vi "Read.vi"(7 "length":u16, 8 "error in (no error)":errorcluster, 9 "Start address":string, 10 "Read Type":variant, 11 "MelsecTCP in":refnum<class "InovanceSerialModbusRtu.lvclass">) -> (0 "error out":errorcluster, 2 "Data":variant, 3 "MelsecTCP out":refnum<class "InovanceSerialModbusRtu.lvclass">)   [LabVIEW 2020, in "HslCommunication.lvlib" / "InovanceSerialModbusRtu.lvclass"]
uses:
  InovanceSerialModbusRtu.lvclass
  D:/Git/Labview-Libraries/Libraries/HslCommunication/Abstract PLC Controler/Abstract PLC Controler.lvclass
  EventLogger.lvlibp/1abvi3w/vi.lib/gpm_packages/@cs/event-logger/Source/Composed Log/Types/Log Level.ctl
  Abstract PLC Controler/Abstract PLC Controler.lvclass/Abstract PLC Controler.ctl
  D:/Git/Labview-Libraries/Libraries/HslCommunication/_Dependenciecs/HslCommunication.dll
  _Dependenciecs/HslCommunication.dll
  Read reference.vi
  Abstract PLC Controler/Abstract PLC Controler.lvclass
  <vilib>/Utility/Data Type/NI_Data Type.lvlib
  EventLogger.lvlibp/Logger.lvclass
  EventLogger.lvlibp/1abvi3w/vi.lib/gpm_packages/@cs/event-logger/Source/Composed Log/Composed Log.lvlib
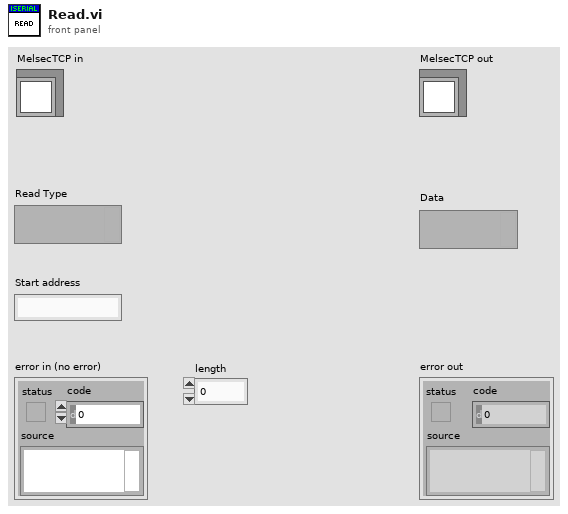
[diagram p1: front panel]
types:
  T1 = typedef "EventLogger.lvlibp/Composed Log.lvlib/Log Level.ctl" = enum16{"Debug", "Info", "Warning", "Error", "Critical"}
  T2 = typedef "NI_Data Type.lvlib/Data Type.ctl" = enum8{"Invalid Type", "Void", "I8", "I16", "I32", "I64", "U8", "U16", "U32", "U64", "Single Float", "Double Float", "Extended Float", "Single Complex", "Double Complex", "Extended Complex", "Enum U8", "Enum U16", "Enum U32", "Enum U64", "Single Float With Unit", "Double Float With Unit", "Extended Float With Unit", "Single Complex with Unit", "Double Complex with Unit", "Extended Complex with Unit", "Boolean", "String", "Path", "Picture", "Tag", "Array", "Cluster", "Variant", "LV Variant", "Waveform", "Timestamp", "Digital Waveform", "Digital Data", "ExpressData", "Refnum", "External Data", "VI", "Poly VI", "LabVIEW Class Instance", "Fixed Point", "Set Collection", "Map Collection"}
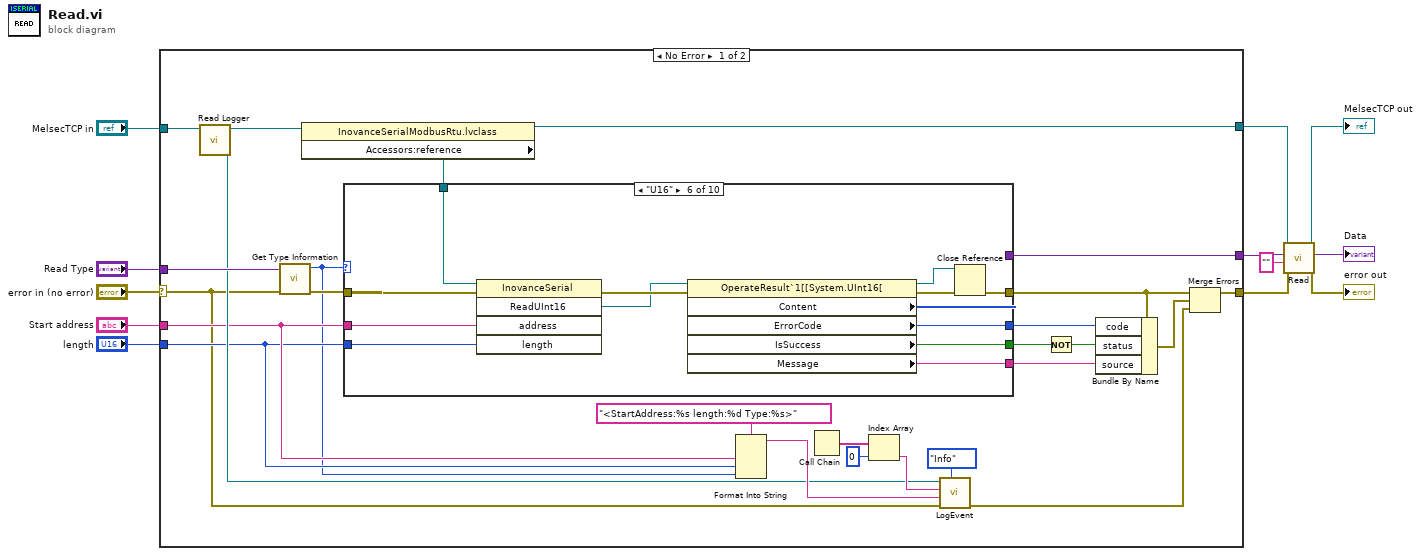
[diagram p0: block diagram]
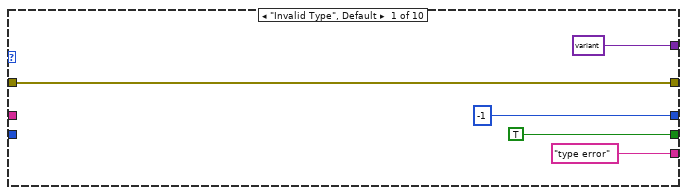
[diagram p2: hidden frame]
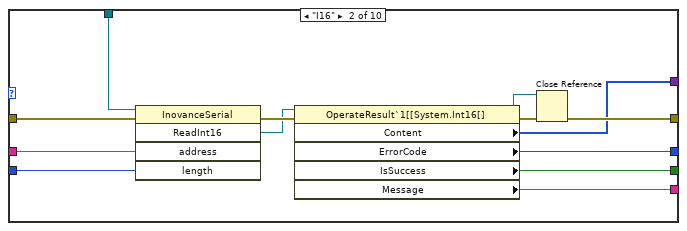
[diagram p3: hidden frame]
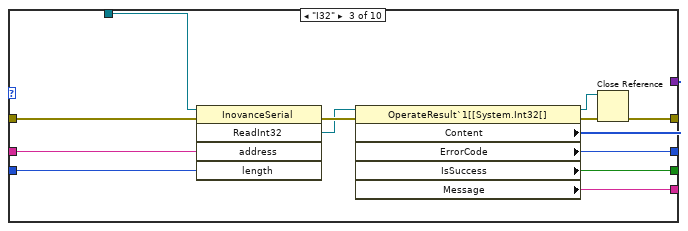
[diagram p4: hidden frame]
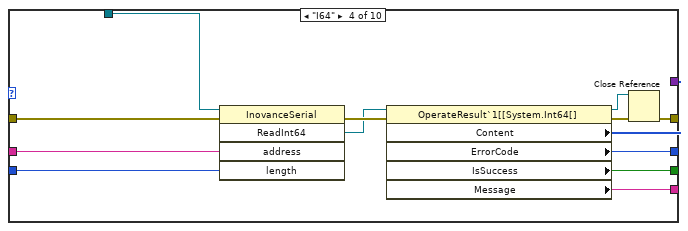
[diagram p5: hidden frame]
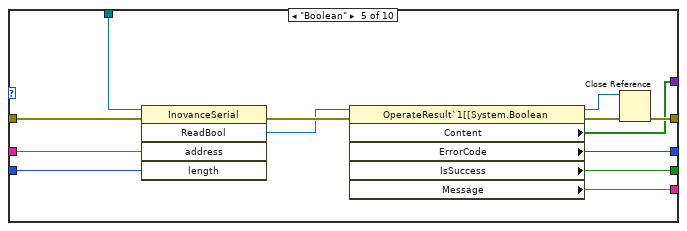
[diagram p6: hidden frame]
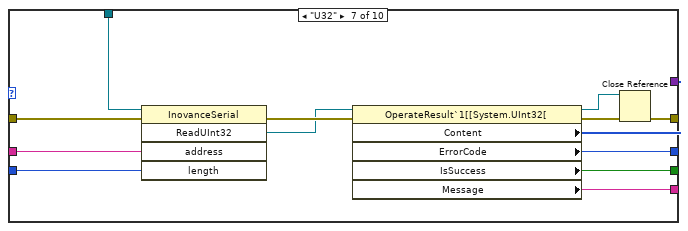
[diagram p7: hidden frame]
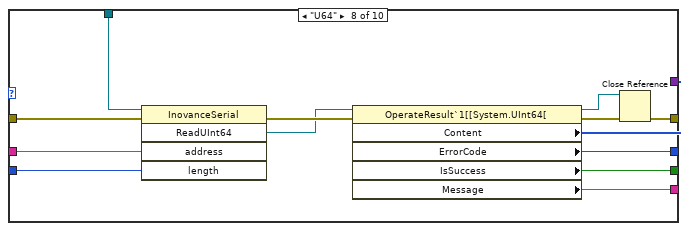
[diagram p8: hidden frame]
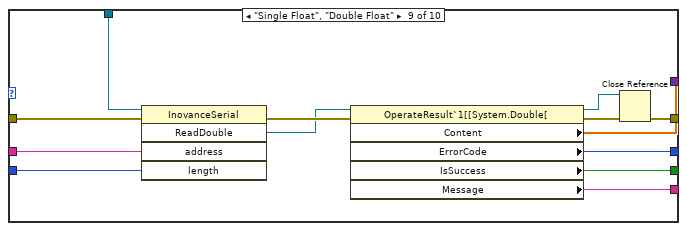
[diagram p9: hidden frame]
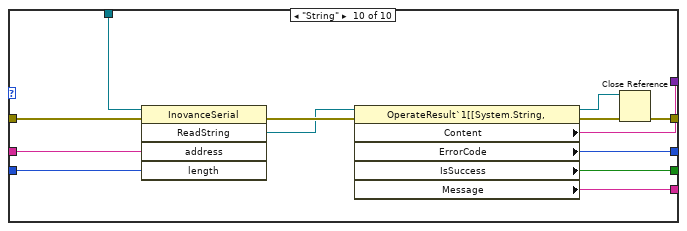
[diagram p10: hidden frame]
diagram:
  n1 = case shown="No Error" "error in (no error)" {
    selector: "error in (no error)" -> [w14 w163]
    tunnel: "MelsecTCP in" -> [w38 w162]
    tunnel: [w29 w162] -> w5
    tunnel: "Start address" -> [w17 _]
    tunnel: [w35 w163] -> w8
    tunnel: [w36 w161] -> w3
    tunnel: "length" -> [w16 _]
    tunnel: "Read Type" -> [w28 w161]
    frame No Error {
      n2 = call "Read Logger.vi"("Abstract PLC Controler in"=w38) -> ("EventLogger.lvlibp:Logger.lvclass"=w19:refnum<class "Logger.lvclass">, "Abstract PLC Controler out"=w20:refnum<class "InovanceSerialModbusRtu.lvclass">)  [unwired: 9 in]
      n3 = call <vilib>:"Get Type Information.vi"("error in (no error)"=w14, "variant"=w28) -> ("error out"=w27:errorcluster, "type"=w15:T2)  [unwired: 5 in, 3 out]
      n4 = property class="InovanceSerialModbusRtu.lvclass"(reference=w20) -> (reference out=w29:refnum<class "InovanceSerialModbusRtu.lvclass">, "Accessors:reference"=w37:refnum<k24>)  [unwired: 1 in, 1 out]
      n5 = case shown="\"U16\"" w15 {
        tunnel: w37 -> [_ w56 w69 w82 w84 w97 w110 w123 w136 w149]
        tunnel: w17 -> [_ w55 w68 w81 w95 w108 w121 w134 w147 w160]
        tunnel: w16 -> [_ w54 w67 w80 w94 w107 w120 w133 w146 w159]
        tunnel: w27 -> [w43 w53 w66 w79 w93 w106 w119 w132 w145 w158]
        tunnel: [w43 w48 w61 w74 w88 w101 w114 w127 w140 w153] -> w31
        tunnel: [variant ("Read Type") w44 w57 w70 w83 w96 w109 w122 w135 w148] -> w36
        tunnel: [-1 ("ErrorCode") w47 w60 w73 w87 w100 w113 w126 w139 w152] -> w34
        tunnel: [TRUE ("IsSuccess") w46 w59 w72 w86 w99 w112 w125 w138 w151] -> w33
        tunnel: ["type error" ("Message") w45 w58 w71 w85 w98 w111 w124 w137 w150] -> w32
        frame "Invalid Type", Default {
        }
        frame "I16" {
          n6 = invoke class="InovanceSerial" method="ReadInt16"(reference=w56, error in=w53, "address"=w55, "length"=w54) -> (error out=w52:errorcluster, "ReadInt16"=w50:refnum<k24>)  [unwired: 1 in, 3 out]
          n7 = property class="OperateResult`1[[System.Int16[]"(reference=w50, error in=w52) -> (reference out=w49:refnum<k24>, error out=w51:errorcluster, "Content"=w44:i16[], "ErrorCode"=w47:i32, "IsSuccess"=w46:bool, "Message"=w45:string)
          n8 = Close Reference(reference=w49, error in (no error)=w51) -> (error out=w48:errorcluster)
        }
        frame "I32" {
          n9 = invoke class="InovanceSerial" method="ReadInt32"(reference=w69, error in=w66, "address"=w68, "length"=w67) -> (error out=w65:errorcluster, "ReadInt32"=w63:refnum<k24>)  [unwired: 1 in, 3 out]
          n10 = property class="OperateResult`1[[System.Int32[]"(reference=w63, error in=w65) -> (reference out=w62:refnum<k24>, error out=w64:errorcluster, "Content"=w57:i32[], "ErrorCode"=w60:i32, "IsSuccess"=w59:bool, "Message"=w58:string)
          n11 = Close Reference(reference=w62, error in (no error)=w64) -> (error out=w61:errorcluster)
        }
        frame "I64" {
          n12 = invoke class="InovanceSerial" method="ReadInt64"(reference=w82, error in=w79, "address"=w81, "length"=w80) -> (error out=w78:errorcluster, "ReadInt64"=w76:refnum<k24>)  [unwired: 1 in, 3 out]
          n13 = property class="OperateResult`1[[System.Int64[]"(reference=w76, error in=w78) -> (reference out=w75:refnum<k24>, error out=w77:errorcluster, "Content"=w70:i64[], "ErrorCode"=w73:i32, "IsSuccess"=w72:bool, "Message"=w71:string)
          n14 = Close Reference(reference=w75, error in (no error)=w77) -> (error out=w74:errorcluster)
        }
        frame "Boolean" {
          n15 = invoke class="InovanceSerial" method="ReadBool"(reference=w84, error in=w93, "address"=w95, "length"=w94) -> (error out=w92:errorcluster, "ReadBool"=w90:refnum<k24>)  [unwired: 1 in, 3 out]
          n16 = property class="OperateResult`1[[System.Boolean"(reference=w90, error in=w92) -> (reference out=w89:refnum<k24>, error out=w91:errorcluster, "Content"=w83:bool[], "ErrorCode"=w87:i32, "IsSuccess"=w86:bool, "Message"=w85:string)
          n17 = Close Reference(reference=w89, error in (no error)=w91) -> (error out=w88:errorcluster)
        }
        frame "U16" {
          n18 = invoke class="InovanceSerial" method="ReadUInt16"(reference=w97, error in=w106, "address"=w108, "length"=w107) -> (error out=w105:errorcluster, "ReadUInt16"=w103:refnum<k24>)  [unwired: 1 in, 3 out]
          n19 = property class="OperateResult`1[[System.UInt16["(reference=w103, error in=w105) -> (reference out=w102:refnum<k24>, error out=w104:errorcluster, "Content"=w96:u16[], "ErrorCode"=w100:i32, "IsSuccess"=w99:bool, "Message"=w98:string)
          n20 = Close Reference(reference=w102, error in (no error)=w104) -> (error out=w101:errorcluster)
        }
        frame "U32" {
          n21 = invoke class="InovanceSerial" method="ReadUInt32"(reference=w110, error in=w119, "address"=w121, "length"=w120) -> (error out=w118:errorcluster, "ReadUInt32"=w116:refnum<k24>)  [unwired: 1 in, 3 out]
          n22 = property class="OperateResult`1[[System.UInt32["(reference=w116, error in=w118) -> (reference out=w115:refnum<k24>, error out=w117:errorcluster, "Content"=w109:u32[], "ErrorCode"=w113:i32, "IsSuccess"=w112:bool, "Message"=w111:string)
          n23 = Close Reference(reference=w115, error in (no error)=w117) -> (error out=w114:errorcluster)
        }
        frame "U64" {
          n24 = invoke class="InovanceSerial" method="ReadUInt64"(reference=w123, error in=w132, "address"=w134, "length"=w133) -> (error out=w131:errorcluster, "ReadUInt64"=w129:refnum<k24>)  [unwired: 1 in, 3 out]
          n25 = property class="OperateResult`1[[System.UInt64["(reference=w129, error in=w131) -> (reference out=w128:refnum<k24>, error out=w130:errorcluster, "Content"=w122:u64[], "ErrorCode"=w126:i32, "IsSuccess"=w125:bool, "Message"=w124:string)
          n26 = Close Reference(reference=w128, error in (no error)=w130) -> (error out=w127:errorcluster)
        }
        frame "Single Float", "Double Float" {
          n27 = invoke class="InovanceSerial" method="ReadDouble"(reference=w136, error in=w145, "address"=w147, "length"=w146) -> (error out=w144:errorcluster, "ReadDouble"=w142:refnum<k24>)  [unwired: 1 in, 3 out]
          n28 = property class="OperateResult`1[[System.Double["(reference=w142, error in=w144) -> (reference out=w141:refnum<k24>, error out=w143:errorcluster, "Content"=w135:dbl[], "ErrorCode"=w139:i32, "IsSuccess"=w138:bool, "Message"=w137:string)
          n29 = Close Reference(reference=w141, error in (no error)=w143) -> (error out=w140:errorcluster)
        }
        frame "String" {
          n30 = invoke class="InovanceSerial" method="ReadString"(reference=w149, error in=w158, "address"=w160, "length"=w159) -> (error out=w157:errorcluster, "ReadString"=w155:refnum<k24>)  [unwired: 1 in, 3 out]
          n31 = property class="OperateResult`1[[System.String,"(reference=w155, error in=w157) -> (reference out=w154:refnum<k24>, error out=w156:errorcluster, "Content"=w148:string, "ErrorCode"=w152:i32, "IsSuccess"=w151:bool, "Message"=w150:string)
          n32 = Close Reference(reference=w154, error in (no error)=w156) -> (error out=w153:errorcluster)
        }
      }
      n33 = Format Into String(format string="<StartAddress:%s length:%d Type:%s>", w17, w16, w15) -> (resulting string=w23:string)  [unwired: 2 in, 1 out]
      n34 = Call Chain() -> (call chain=w26:string[])
      n35 = Index Array(array=w26, index=0) -> (element=w22:string)
      n36 = call "LogEvent.vi"("Event Level"=Log_Level."Info", "error in (no error)"=w14, "Data To Log"=w23, "SourceID"=w22, "Logger in"=w19) -> ("error out"=w18:errorcluster)  [unwired: 5 in, 1 out]
      n37 = Not(x=w33) -> (.not. x?=w13:bool)
      n38 = Bundle By Name(cluster=w31, "code"=w34, "status"=w13, "source"=w32) -> (w30:errorcluster)
      n39 = Merge Errors(w31, w30, w18) -> (w35:errorcluster)
    }
    frame Error {
    }
  }
  n40 = call-parent "Read.vi"("error in (no error)"=w8, "Start address"="", "Read Type"=w3, "MelsecTCP in"=w5) -> ("error out"=→"error out":errorcluster, "Data"=→"Data":variant, "MelsecTCP out"=→"MelsecTCP out":refnum<class "InovanceSerialModbusRtu.lvclass">)  [unwired: 5 in]
